vi "create.all.vi"() -> (3 "all":refnum<class "all.lvclass">)   [LabVIEW 2020, in "nominal types.lvlib" / "channelFilter.lvlib" / "channelFilter.lvclass"]
uses:
  channelFilter.lvclass
  all/all.lvclass
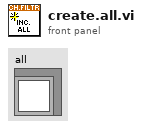
[diagram p1: front panel]
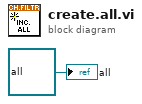
[diagram p0: block diagram]
diagram:
  "all" <- refnum<class "all.lvclass"> refnum ("nominal types.lvlib:channelFilter.lvlib:all.lvclass")
